vi "Compare With Previous.vi"(3 "Variant":variant) -> (1 "Not Equal?":bool)   [LabVIEW 2016, in "Control Experiment SM.lvclass"]
uses:
  Control Experiment SM.lvclass
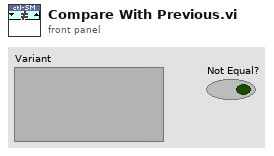
[diagram p1: front panel]
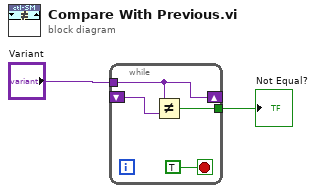
[diagram p0: block diagram]
diagram:
  n1 = while {
    shift-right: [w5] -> _
    shift-left: _ -> [w3]
    tunnel: "Variant" -> [w5]
    tunnel: [w4] -> w2
    stop <- TRUE stop-if-true
    n2 = Not Equal?(x=w5, y=w3) -> (x != y?=w4:bool)
  }
  "Not Equal?" <- w2
